vi "Write to Hardware.vi"(7 "valid triggers":bool, 8 "error in":errorcluster, 9 "trigger values":dbl[](array[numeric]), 10 "Values in":dbl[](array[numeric]), 11 "Ballard ARINC-429 Tx Acyclic execution unit in":refnum<class "Tx Acyclic Labels Execution Unit.lvclass">) -> (0 "error out":errorcluster, 1 "trigger values out":dbl[](array[numeric]), 2 "Values out":dbl[](array[numeric]), 3 "Ballard ARINC-429 Tx Acyclic execution unit out":refnum<class "Tx Acyclic Labels Execution Unit.lvclass">)   [LabVIEW 2023, in "Ballard ARINC 429 Engine.lvlib" / "Implementation.lvlib" / "Tx Acyclic Labels Execution Unit.lvclass"]
uses:
  Tx Acyclic Labels Execution Unit.lvclass
  Tx Acyclic Labels Execution Unit.lvclass/Tx Acyclic Labels Execution Unit.ctl
  Shared/Encode Parameter and Update Word (32-bit).vi/1445f95d-237d-4fc6-96b9-8992d347f513.vi
  Shared/Encode Parameter and Update Word (32-bit).vi/6b8853f0-8e5d-49e3-9391-4d3f8e5314b0.vi
  Shared/Encode Parameter and Update Word (32-bit).vi/2babc4f4-546e-4d35-846d-a4a1fbac0249.vi
  Custom Device/Write Error to System Log.vi/ca55ed61-c1f5-4d13-8aef-490b87d2cf89.vi
  Shared/Encode Parameter and Update Word (32-bit).vi/1445f95d-237d-4fc6-96b9-8992d347f513.vi/9377bb8f-44b5-4a8f-87f1-966fd5a9edcc.vi
  Shared/Encode Parameter and Update Word (32-bit).vi/1445f95d-237d-4fc6-96b9-8992d347f513.vi/e95d9d1f-307c-44d6-9f26-c3f519a4990d.vi
  Shared/Encode Parameter and Update Word (32-bit).vi/1445f95d-237d-4fc6-96b9-8992d347f513.vi/0c23f515-4369-4514-bc3d-4444e6b437b2.vi
  Shared/Encode Parameter and Update Word (32-bit).vi/6b8853f0-8e5d-49e3-9391-4d3f8e5314b0.vi/136dcdcb-2dd3-4a4d-a796-a8f7a3f8e1ac.vi
  Shared/Encode Parameter and Update Word (32-bit).vi/6b8853f0-8e5d-49e3-9391-4d3f8e5314b0.vi/a54b505c-1216-4ef4-8378-3ceda9d188df.vi
  <vilib>/NI/NI VeriStand Encoding and Decoding/Get Bits Per Digit from Base.vi
  <vilib>/NI VeriStand/Custom Device Tools/Custom Device Utility Library/NI VeriStand - Print Debug Line.vi
  Custom Device/Custom Device.lvlib
  Hardware API/Ballard ARINC 429 Hardware API.lvlib
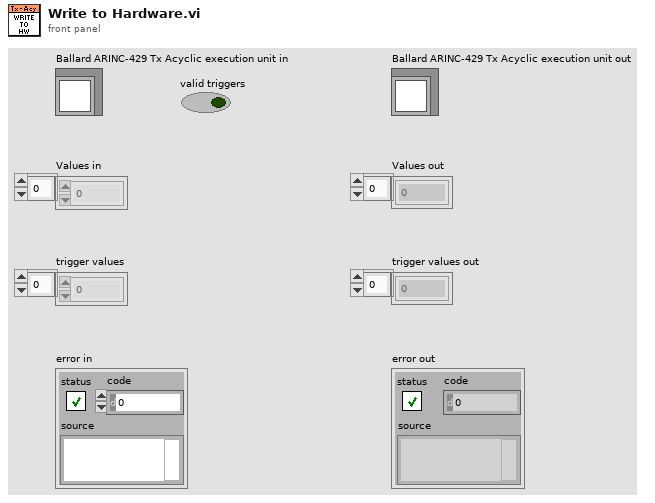
[diagram p1: front panel]
types:
  T1 = typedef "RT Hardware Channel Settings.ctl" = cluster{"channel #":u16, "channel handle":u64, "labels settings for RT":T2[]}
  T2 = typedef "RT Label Settings.ctl" = cluster{"Name":string, "xmlName":string, "label":T3, "transfer period":u32, "SDI_Enabled":bool, "SDI":u8, "parameter driver data":T4, "transfer type":T8, "has timestamp?":bool, "Label Disable/Trigger Channel Reference":T7, "Message Handle":u64, "Initialized?":bool, "Word Initial Raw Value":u32, "Label Timestamp Channel Data Reference":T9, "disabled":bool}
  T3 = typedef "Label.ctl" = u8
  T4 = typedef "RT Parameters.ctl" = cluster{"parameter definitions":T5[], "Tx parameter refs":T7[]}
  T5 = typedef "Parameter Definition.ctl" = cluster{"start index":i32, "size":i32, "encoding":T6, "signed":bool, "scale multiplier":dbl, "scale offset":dbl}
  T6 = typedef "Encoding and Decoding.lvlib/Encoding.ctl" = enum16{"BNR", "BCD", "Discrete"}
  T7 = typedef "Custom Device API.lvlib/Custom Device Item Ref.ctl" = u64
  T8 = typedef "Transfer Type.ctl" = enum16{"Scheduled", "Acyclic", "Block", "Strobe"}
  T9 = typedef "Custom Device API.lvlib/Data Reference.ctl" = i32
  T10 = typedef "Map of Values Indexes to Channel and Label Indexes.ctl" = map{i32, cluster{"channel index":i32, "label index":i32, "group values start index":i32, "values in group":i32}}
  T11 = cluster{"channel index":i32, "label index":i32, "group values start index":i32, "values in group":i32}
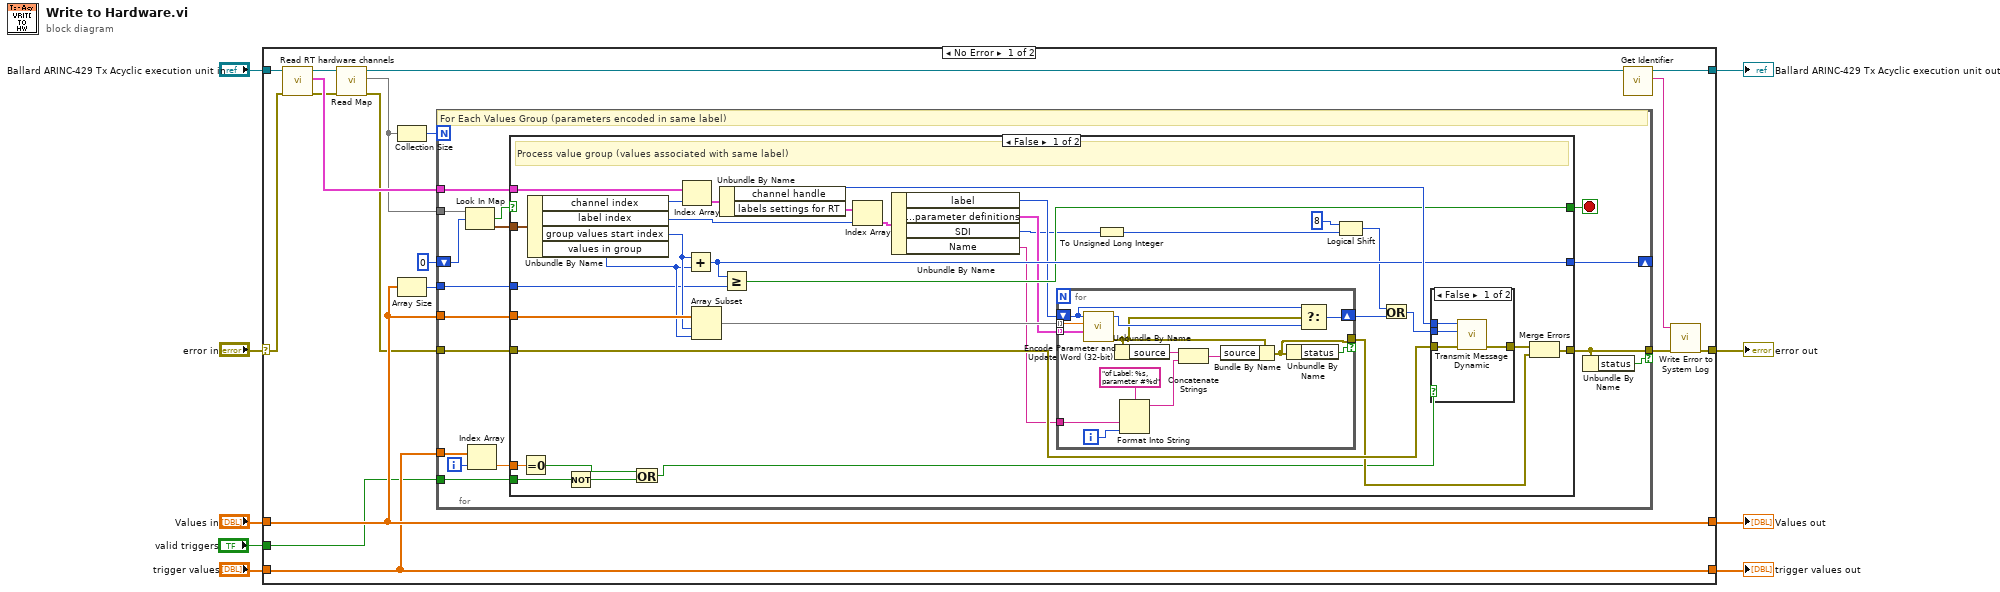
[diagram p0: block diagram]
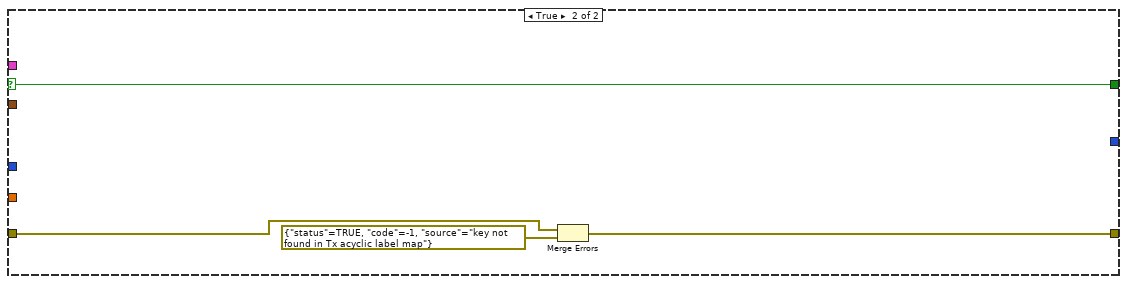
[diagram p3: hidden frame]
diagram:
  n1 = case shown="No Error" "error in" {
    selector: "error in" -> [w21 w102]
    tunnel: [w11 w102] -> w9
    tunnel: [w23 w101] -> w7
    tunnel: "Values in" -> [w23 w101]
    tunnel: [w14 w103] -> w5
    tunnel: "Ballard ARINC-429 Tx Acyclic execution unit in" -> [w20 w103]
    tunnel: "trigger values" -> [w16 w100]
    tunnel: [w16 w100] -> w2
    tunnel: "valid triggers" -> [w10 _]
    frame No Error {
      n2 = call "Read RT hardware channels.vi"("error in"=w21, "Ballard ARINC-429 Tx Acyclic execution unit in"=w20) -> ("error out"=w18:errorcluster, "RT hardware channels"=w27:T1[], "Ballard ARINC-429 Tx Acyclic execution unit out"=w19:refnum<class "Tx Acyclic Labels Execution Unit.lvclass">)  [unwired: 7 in]
      n3 = call "Read Map.vi"("error in"=w18, "Ballard ARINC-429 Tx Acyclic execution unit in"=w19) -> ("error out"=w17:errorcluster, "map from values indexes to RT info indexes"=w24:T10, "Ballard ARINC-429 Tx Acyclic execution unit out"=w15:refnum<class "Tx Acyclic Labels Execution Unit.lvclass">)  [unwired: 7 in]
      n4 = Collection Size(1:w24) -> (0:w25:i32)
      n5 = Array Size(array=w23) -> (size(s)=w22:i32)
      n6 = for {
        N: w25 -> [_]
        tunnel: w23 -> [w38]
        tunnel: w24 -> [w41]
        shift-right: [w37] -> _
        shift-left: 0 -> [w40]
        tunnel: w17 -> [w43]
        tunnel: [w33] -> w12 if=w32
        tunnel: w22 -> [w35]
        tunnel: w27 -> [w42]
        tunnel: w16 -> [w30]
        tunnel: w10 -> [w28]
        i -> [w31]
        stop <- w34 stop-if-true
        # "For Each Values Group (parameters encoded in same label)"
        n7 = Look In Map(map=w41, key=w40) -> (key not found?=w36:bool, value=w39:T11)  [unwired: 1 in]
        n8 = Index Array(array=w30, index=w31) -> (element=w29:dbl)
        n9 = case shown="False" w36 {
          selector: w36 -> [_ w96]
          tunnel: w43 -> [w61 w99]
          tunnel: [w60 w97] -> w33
          tunnel: w42 -> [w66 _]
          tunnel: w39 -> [w76 _]
          tunnel: w38 -> [w75 _]
          tunnel: [w64 _] -> w37
          tunnel: w35 -> [w63 _]
          tunnel: [w62 w96] -> w34
          tunnel: w29 -> [w59 _]
          tunnel: w28 -> [w52 _]
          frame False {
            # "Process value group (values associated with same label)"
            n10 = Equal To 0?(x=w59) -> (x = 0?=w54:bool)
            n11 = Unbundle By Name(w76) -> ("channel index"=w69:i32, "label index"=w70:i32, "group values start index"=w74:i32, "values in group"=w73:i32)
            n12 = Not(x=w52) -> (.not. x?=w51:bool)
            n13 = Or(x=w54, y=w51) -> (x .or. y?=w53:bool)
            n14 = Index Array(array=w66, index=w69) -> (element=w68:T1)
            n15 = Add(x=w74, y=w73) -> (x+y=w64:i32)
            n16 = Array Subset(array=w75, index=w74, length=w73) -> (w72:dbl[])
            n17 = Unbundle By Name(w68) -> ("channel handle"=w65:u64, "labels settings for RT"=w67:T2[])
            n18 = Greater Or Equal?(x=w64, y=w63) -> (x >= y?=w62:bool)
            n19 = Index Array(array=w67, index=w70) -> (element=w71:T2)
            n20 = Unbundle By Name(w71) -> ("label"=w57:T3, "parameter driver data.parameter definitions"=w58:T5[], "SDI"=w48:u8, "Name"=w44:string)
            n21 = for {
              tunnel: w72 -> [w90] mode=indexing
              shift-right: [w85] -> w50
              shift-left: w57 -> [w88]
              tunnel: w58 -> [w89] mode=indexing
              tunnel: [w79] -> w55 if=w87
              tunnel: w44 -> [w78]
              i -> [w77]
              n22 = call "Encode Parameter and Update Word (32-bit).vi"("parameter definition"=w89, "parameter value"=w90, "word in"=w88) -> ("error out"=w80:errorcluster, "word out"=w86:u32)  [unwired: 7 in]
              n23 = Unbundle By Name(w80) -> ("source"=w84:string)
              n24 = Format Into String(format string="of Label: %s, parameter #%d", w78, w77) -> (resulting string=w81:string)  [unwired: 2 in, 1 out]
              n25 = Concatenate Strings(w84, w81) -> (w83:string)
              n26 = Bundle By Name(cluster=w80, "source"=w83) -> (w79:errorcluster)
              n27 = Unbundle By Name(w79) -> ("status"=w87:bool)
              n28 = Select(t=w88, s=w80, f=w86) -> (s? t:f=w85:u32)
            }
            n29 = To Unsigned Long Integer(number=w48) -> (unsigned 32bit integer=w45:u32)
            n30 = Logical Shift(y=i16 8, x=w45) -> (x << y=w47:u32)
            n31 = Or(x=w47, y=w50) -> (x .or. y?=w49:u32)
            n32 = case shown="False" w53 {
              tunnel: w65 -> [w94 _]
              tunnel: w61 -> [w93 w95]
              tunnel: w49 -> [w92 _]
              tunnel: [w91 w95] -> w56
              frame False {
                n33 = call "Transmit Message Dynamic.vi"("error in (no error)"=w93, "message data"=w92, "channel handle in"=w94) -> ("error out"=w91:errorcluster)  [unwired: 7 in, 1 out]
              }
              frame True {
              }
            }
            n34 = Merge Errors(w56, w55) -> (w60:errorcluster)
          }
          frame True {
            n35 = Merge Errors(w99, errorcluster {"status"=TRUE, "code"=-1, "source"="key not found in Tx acyclic label map"} ("error in")) -> (w97:errorcluster)
          }
        }
        n36 = Unbundle By Name(w33) -> ("status"=w32:bool)
      }
      n37 = call-dynamic "Get Identifier.vi"("Ballard ARINC-429 Execution Unit in"=w15) -> ("identifier"=w13:string, "Ballard ARINC-429 Execution Unit out"=w14:refnum<class "Tx Acyclic Labels Execution Unit.lvclass">)  [unwired: 8 in, 1 out]
      n38 = call "Write Error to System Log.vi"("error in"=w12, "identifier"=w13) -> ("error out"=w11:errorcluster)  [unwired: 9 in]
    }
    frame Error {
    }
  }
  "error out" <- w9
  "Ballard ARINC-429 Tx Acyclic execution unit out" <- w5
  "Values out" <- w7
  "trigger values out" <- w2
